vi "Main.vi"(11 "Module Admin":refnum<class "Delacor_lib_QMH_Module Admin.lvclass">) -> ()   [LabVIEW 2020, in "Cycling by Event module.lvlib"]
doc: "This template is based off of the Queued Message Handler design pattern and the Queued Message Handler project template that ships with LabVIEW.\n\nThe main difference is that the queue is private to this module and communication between modules is performed via Broadcast and Request events.\n\nRequest events are wrapped in public API methods and are handled in the Event Handling Loop (EHL) of this VI. Any module can register for Broadcast events sent by this module. The EHL generates messages based on user interface actions.\n\nThe Message Handling Loop (MHL) processes messages generated by the EHL, or by other messages. The messages are string values, so new messages can be added easily to the Message Cases case structure in the MHL. Each message cluster can also provide an optional value for Message Data, which is a variant that can be converted to whatever message-specific data is required.\n_____\nBased on DQMH Project Template 7.0.1.1316."
uses:
  Cycling by Event module.lvlib
  <vilib>/Delacor/Delacor QMH/Libraries/Module Admin_class/Delacor_lib_QMH_Module Admin.lvclass
  Module Data--cluster.ctl
  RPM updated HL Data--cluster.ctl
  Cycling by State module/Cycling state.ctl
  <vilib>/Delacor/Delacor QMH/Libraries/Message Queue_class/Delacor_lib_QMH_Message Queue.lvclass/Delacor_lib_QMH_Message Queue.ctl
  Stop Argument--cluster.ctl
  <vilib>/Delacor/Delacor QMH/Libraries/Module Admin_class/Delacor_lib_QMH_Module Admin.lvclass/Delacor_lib_QMH_Module Admin.ctl
  Start cycling Argument--cluster.ctl
  Detecting 110rpm Argument--cluster.ctl
  Detecting 100rpm Argument--cluster.ctl
  Detecting 0rpm Argument--cluster.ctl
  Stop cycling Argument--cluster.ctl
  <vilib>/Utility/miscctls.llb/LVPointTypeDef.ctl
  <vilib>/Delacor/Delacor QMH/Libraries/Message Queue_class/Delacor_lib_QMH_Enqueue Message (Single).vi
  <vilib>/Delacor/Delacor QMH/Libraries/Module Admin_class/Delacor_lib_QMH_Get External Launch.vi
  <vilib>/Delacor/Delacor QMH/Libraries/Message Queue_class/Delacor_lib_QMH_Message Queue.lvclass
  Sensor checking module/Sensor checking module.lvlib
panel:
  out "error out":errorcluster
  out "Status":string
  in  "Simulate MHL Error":bool
  in  "Simulate EHL Error":bool
  # "Other processes communicate with this Module via its Public API (wrappers for its Request Events).\n\nThis Module communicates with other processes via its Broadcast Events.\nAny process that wants to receive these messages can register for this module's Broadcast events."
  # "This template is for the DQMH framework. See the block diagram for more information on how to use this template."
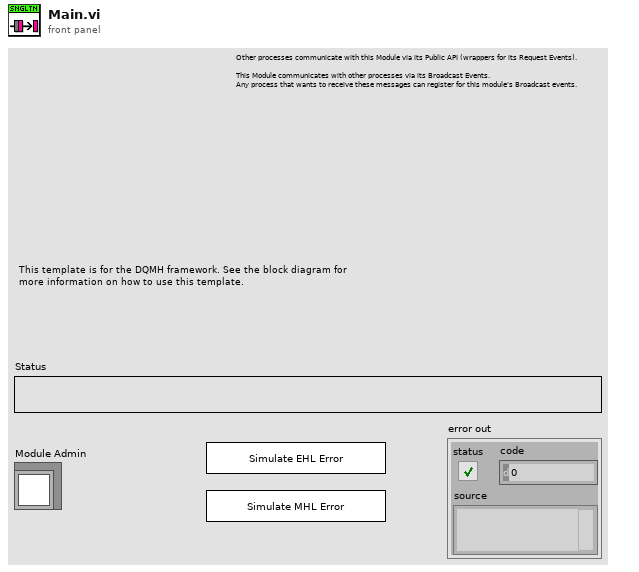
[diagram p1: front panel]
types:
  T1 = typedef "Cycling by Event module.lvlib/Request Events--cluster.ctl" = cluster{"Stop Module":refnum<user-event>, "Show Panel":refnum<user-event>, "Hide Panel":refnum<user-event>, "Get Module Execution Status":refnum<user-event>, "Show Diagram":refnum<user-event>, "Start cycling":refnum<user-event>, "Detecting 110rpm":refnum<user-event>, "Change state to HL":refnum<user-event>, "Detecting 100rpm":refnum<user-event>, "Detecting 0rpm":refnum<user-event>, "Stop cycling":refnum<user-event>}
  T2 = typedef "Sensor checking module.lvlib/Broadcast Events--cluster.ctl" = cluster{"Module Did Init":refnum<user-event>, "Status Updated":refnum<user-event>, "Error Reported":refnum<user-event>, "Module Did Stop":refnum<user-event>, "Update Module Execution Status":refnum<user-event>, "Triggered Broadcast":refnum<user-event>}
  T3 = typedef "Cycling by Event module.lvlib/RPM updated HL Data--cluster.ctl" = cluster{"Enum":T4}
  T4 = typedef "Cycling state.ctl" = enum16{"Accelerating to 110rpm", "Detecting 100rpm", "Pressing until 0rpm"}
  T5 = typedef "Cycling by Event module.lvlib/Module Data--cluster.ctl" = cluster{"Status":string, "Triggered interval":dbl}
  T6 = enum32{"invalid lock state", "Not Locked", "Locked (No Password)", "Password-protected"}
  T7 = typedef "Cycling by Event module.lvlib/Stop Argument--cluster.ctl" = cluster{"Origin":string, "Exit via Stop Module Req?":bool, "Wait for Module to stop?":bool}
  T8 = typedef "Cycling by Event module.lvlib/Start cycling Argument--cluster.ctl" = cluster{"Triggered interval":dbl}
  T9 = typedef "Cycling by Event module.lvlib/Detecting 110rpm Argument--cluster.ctl" = cluster{"RPM":dbl}
  T10 = typedef "Cycling by Event module.lvlib/Detecting 100rpm Argument--cluster.ctl" = cluster{"RPM":dbl}
  T11 = typedef "Cycling by Event module.lvlib/Detecting 0rpm Argument--cluster.ctl" = cluster{"RPM":dbl}
  T12 = typedef "Cycling by Event module.lvlib/Stop cycling Argument--cluster.ctl" = cluster{"Boolean":bool}
  T13 = typedef "LVPointTypeDef.ctl" = cluster{"Horizontal":i16, "Vertical":i16}
  T14 = enum32{"Invalid", "Standard", "Closed", "Hidden", "Minimized", "Maximized"}
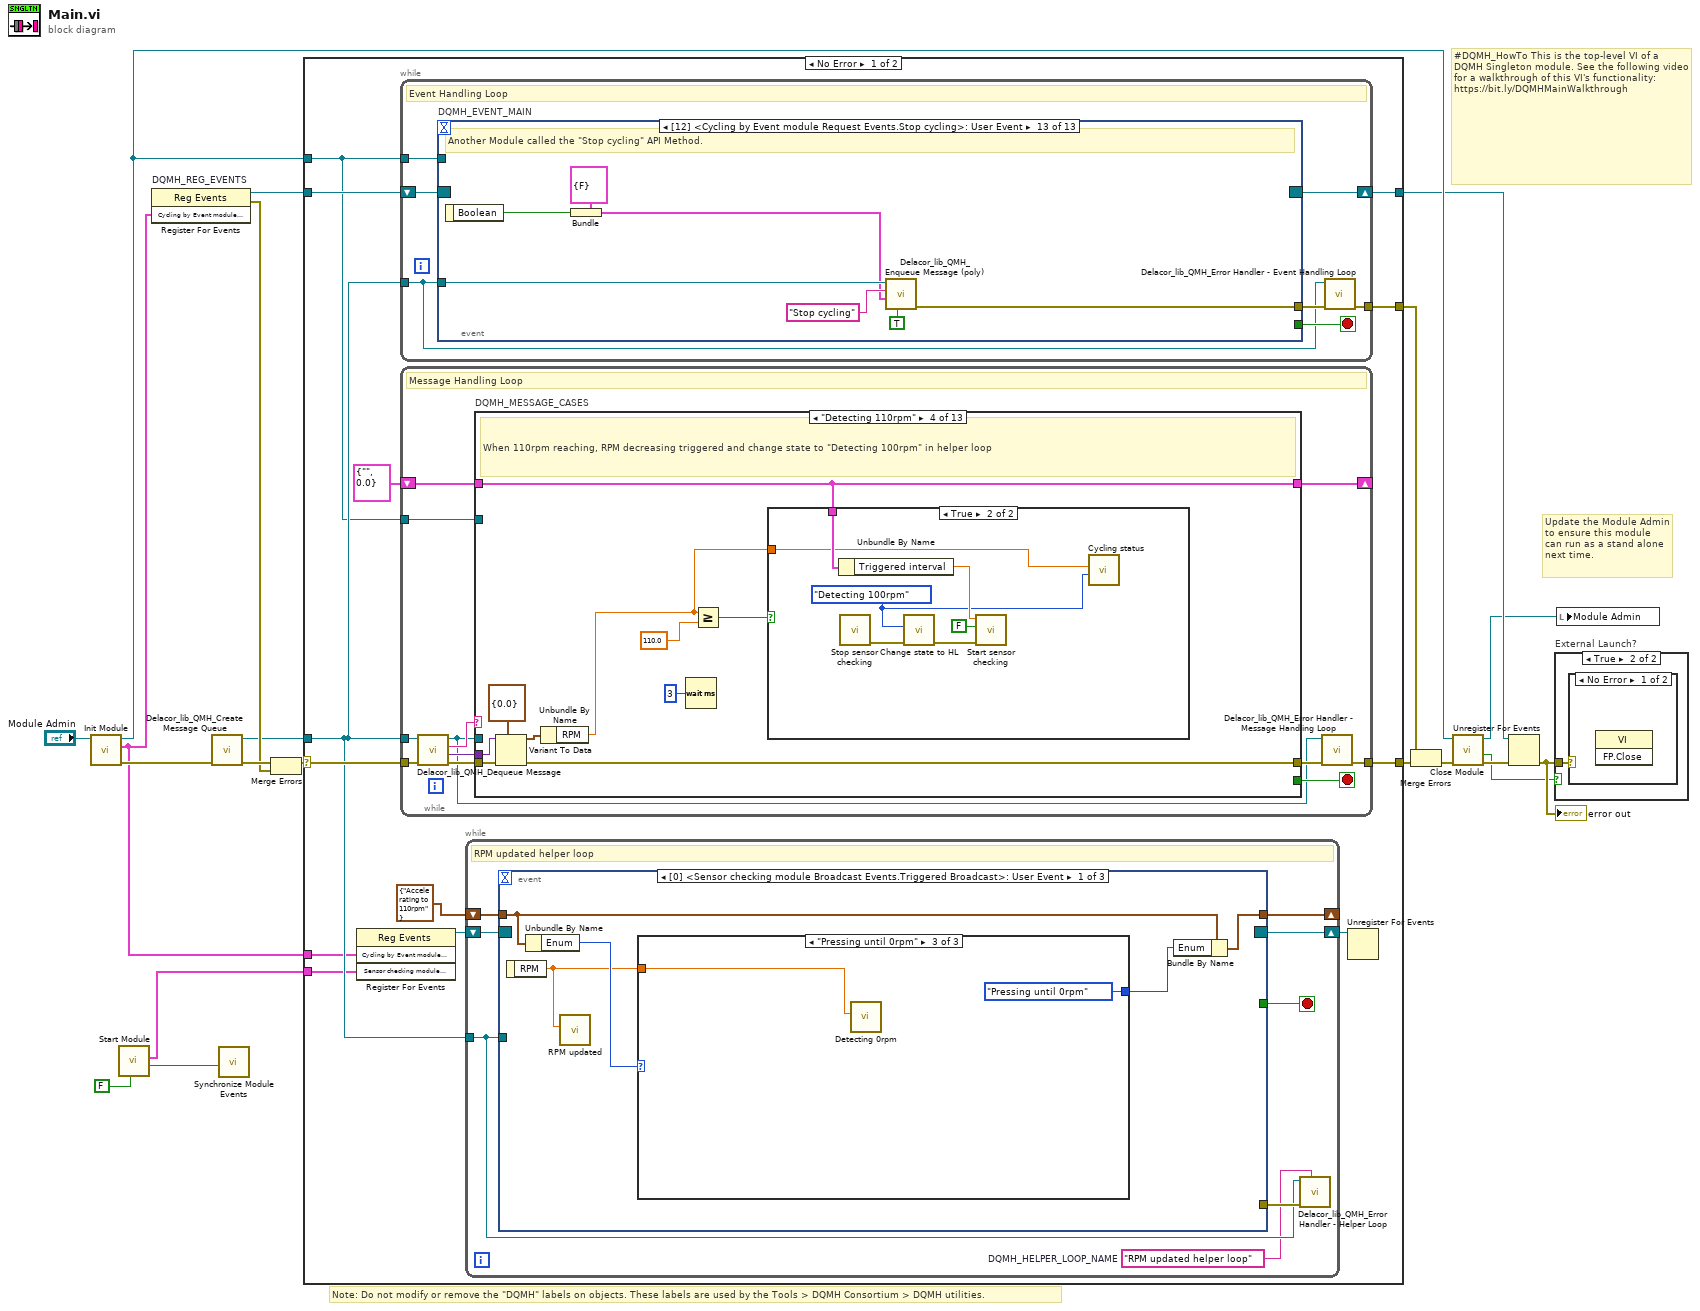
[diagram p0: block diagram]
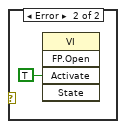
[diagram p3: hidden frame]
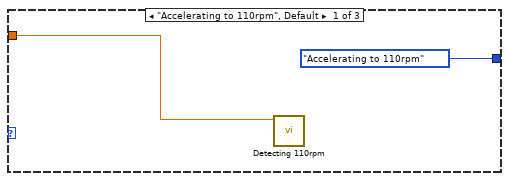
[diagram p4: hidden frame]
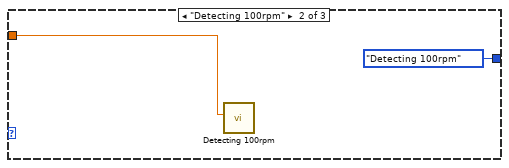
[diagram p5: hidden frame]
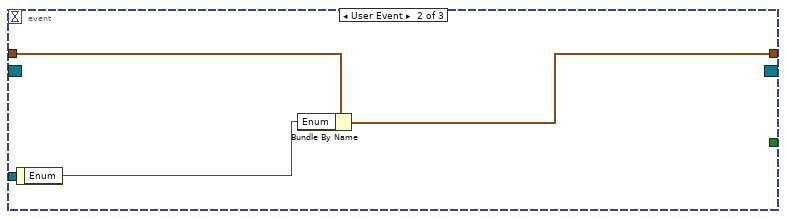
[diagram p6: hidden frame]
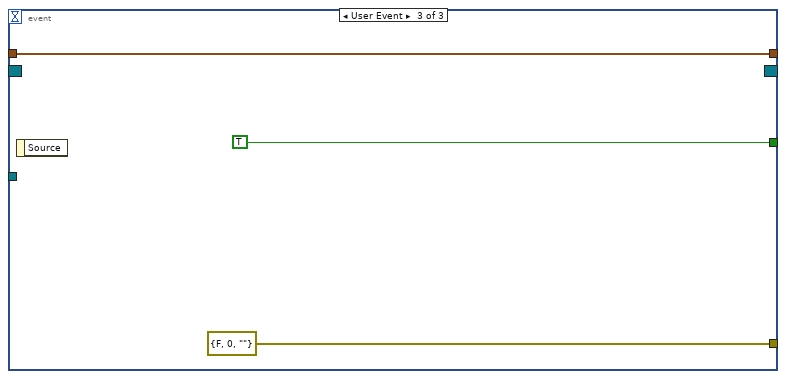
[diagram p7: hidden frame]
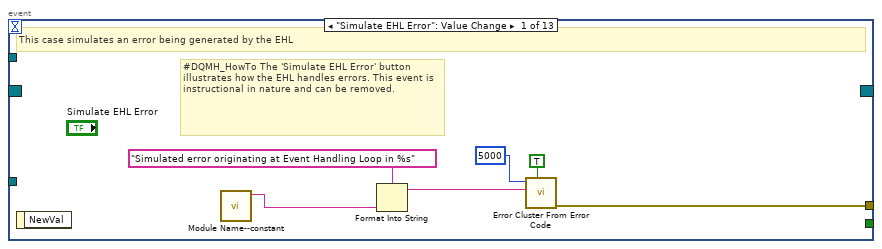
[diagram p8: hidden frame]
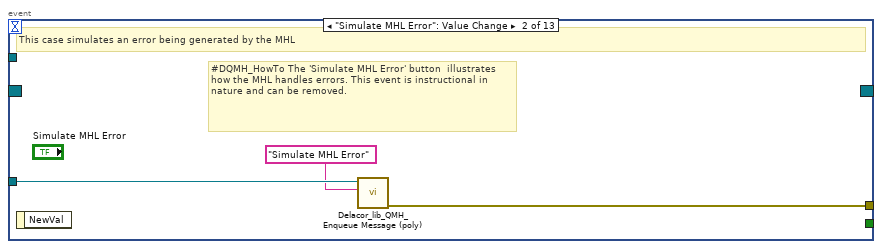
[diagram p9: hidden frame]
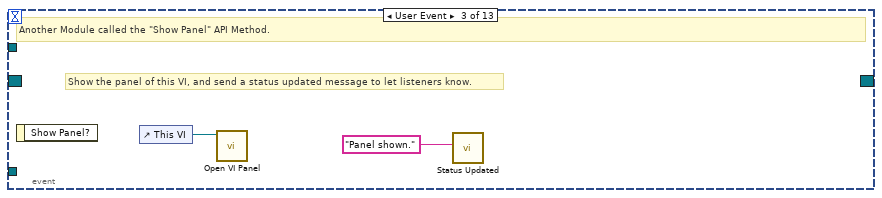
[diagram p10: hidden frame]
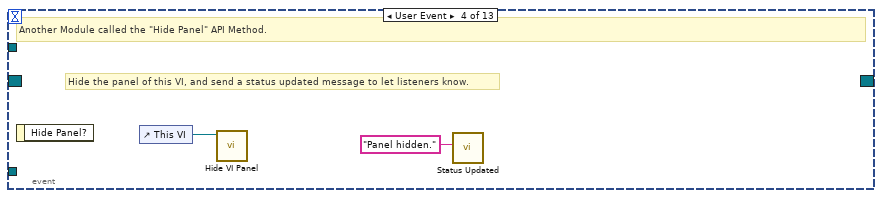
[diagram p11: hidden frame]
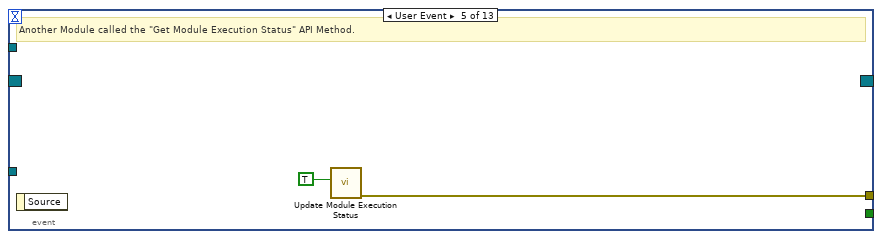
[diagram p12: hidden frame]
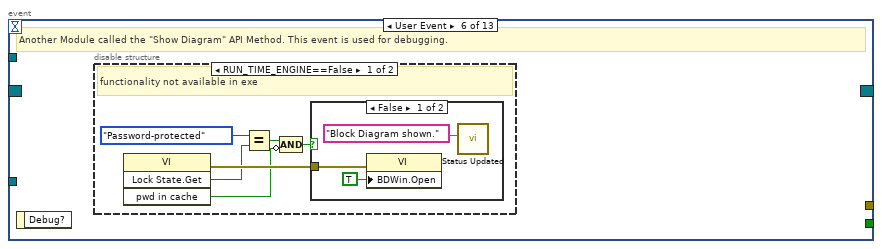
[diagram p13: hidden frame]
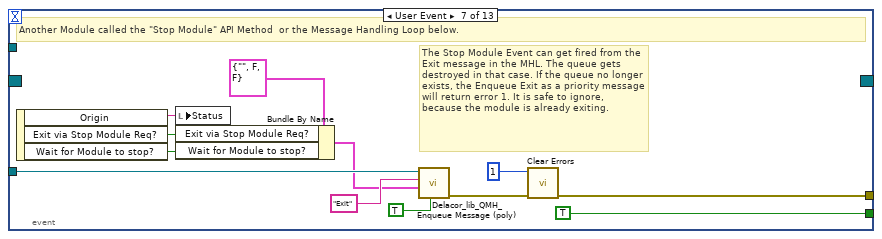
[diagram p16: hidden frame]
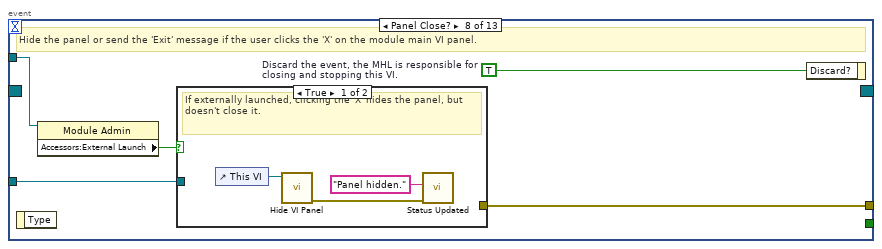
[diagram p17: hidden frame]
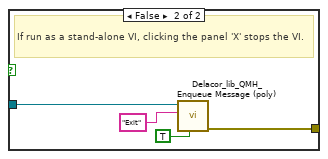
[diagram p18: hidden frame]
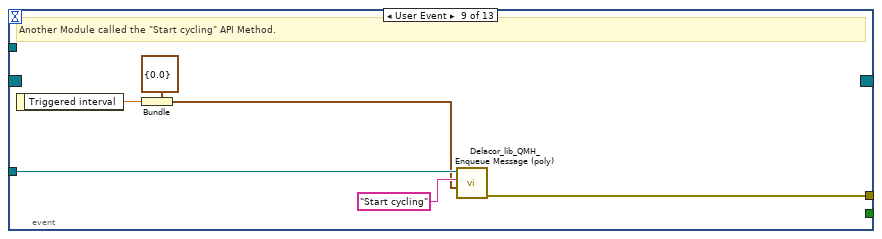
[diagram p19: hidden frame]
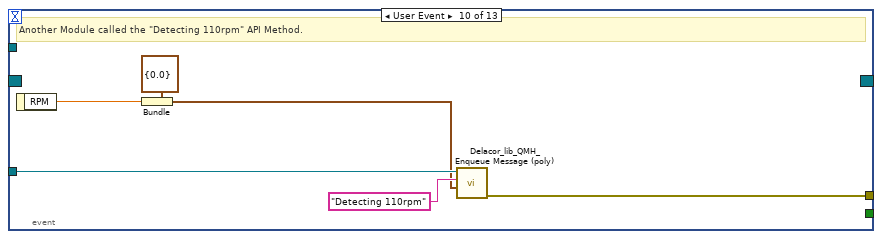
[diagram p20: hidden frame]
diagram:
  # "#DQMH_HowTo This is the top-level VI of a DQMH Singleton module. See the following video for a walkthrough of this VI's functionality: https://bit.ly/DQMHMainWalkthrough"
  # "Note: Do not modify or remove the \"DQMH\" labels on objects. These labels are used by the Tools > DQMH Consortium > DQMH utilities."
  # "Update the Module Admin to ensure this module can run as a stand alone next time."
  n1 = call "Init Module.vi"("Singleton Module Admin in"="Module Admin") -> ("error out"=w19:errorcluster, "Cycling by Event module Request Events"=w4:T1, "Singleton Module Admin out"=w11:refnum<class "Delacor_lib_QMH_Module Admin.lvclass">)  [unwired: 8 in]
  n2 = call "Start Module.vi"("Show Main VI Diagram on Init (F)"=FALSE) -> ("Wait for Event Sync?"=w3:bool, "Sensor checking module Broadcast Events"=w1:T2)  [unwired: 7 in, 2 out]
  n3 = register-events "DQMH_REG_EVENTS"(w4) -> (reference out=w9:refnum<event-registration>, error out=w12:errorcluster)  [unwired: 2 in]
  n4 = call <vilib>:"Delacor_lib_QMH_Create Message Queue.vi"("error in"=w19) -> ("error out"=w14:errorcluster, "Message Queue"=w8:refnum<class "Delacor_lib_QMH_Message Queue.lvclass">)  [unwired: 9 in]
  n5 = call "Synchronize Module Events.vi"("Wait for Event Sync?"=w3) -> ()  [unwired: 10 in, 1 out]
  n6 = Merge Errors(w14, w12) -> (w13:errorcluster)
  n7 = case shown="No Error" w13 {
    selector: w13 -> [w31 w303]
    tunnel: [w33 w302] -> w20
    tunnel: [w30 w301] -> w10
    tunnel: w9 -> [w28 w301]
    tunnel: w8 -> [w27 w296]
    tunnel: [w32 _] -> w17
    tunnel: w11 -> [w26 w297]
    tunnel: w4 -> [w25 _]
    tunnel: w1 -> [w22 _]
    frame No Error {
      n8 = register-events ("DQMH_HELPER_REGFOREVENTS")(w25, w22) -> (reference out=w23:refnum<event-registration>)  [unwired: 2 in, 1 out]
      n9 = while {
        tunnel: w27 -> [w59]
        shift-right: [w62] -> w30
        shift-left: w28 -> [w63]
        tunnel: [w64] -> w32
        tunnel: w26 -> [w60]
        stop <- w61 stop-if-true
        # "Event Handling Loop"
        n10 = event "DQMH_EVENT_MAIN" shown="[12] <Cycling by Event module Request Events.Stop cycling>: User Event" {
          selector: w63 -> [_ _ _ _ _ _ _ _ _ _ _ _ _]
          dyn-events: [_ _ _ _ _ _ _ _ _ _ _ _ _] -> w62
          timeout: _ -> [_ _ _ _ _ _ _ _ _ _ _ _ _]
          tunnel: [_ _ _ _ _ _ TRUE ("Discard?") _ _ _ _ _ _] -> w61
          tunnel: w59 -> [_ w73 _ _ _ _ w97 w104 w119 w125 w131 w137 w144]
          tunnel: [w71 w74 _ _ w80 _ w100 w106 w114 w120 w126 w132 w139] -> w65
          tunnel: w60 -> [_ _ _ _ _ _ _ w103 _ _ _ _ _]
          event "Simulate EHL Error": Value Change {
            # "#DQMH_HowTo The 'Simulate EHL Error' button  illustrates how the EHL handles errors. This event is instructional in nature and can be removed."
            # "This case simulates an error being generated by the EHL"
            n11 = event-data() -> ()  [unwired: 1 in, 1 out]
            n12 = call "Module Name--constant.vi"() -> ("Module Name"=w68:string)  [unwired: 11 in]
            n13 = Format Into String(format string="Simulated error originating at Event Handling Loop in %s", w68) -> (resulting string=w69:string)  [unwired: 2 in, 1 out]
            n14 = call <vilib>:"Error Cluster From Error Code.vi"("show call chain? (False)"=TRUE, "error message (\"\")"=w69, "error code (0)"=5000) -> ("error out"=w71:errorcluster)  [unwired: 6 in]
          }
          event "Simulate MHL Error": Value Change {
            # "#DQMH_HowTo The 'Simulate MHL Error' button  illustrates how the MHL handles errors. This event is instructional in nature and can be removed."
            # "This case simulates an error being generated by the MHL"
            n15 = event-data() -> ()  [unwired: 1 in, 1 out]
            n16 = call-poly <vilib>:"Delacor_lib_QMH_Enqueue Message (poly).vi"("Message"="Simulate MHL Error", "Message Queue in"=w73) -> ("error out"=w74:errorcluster)  [unwired: 8 in, 1 out]
          }
          event User Event {
            # "Show the panel of this VI, and send a status updated message to let listeners know."
            # "Another Module called the \"Show Panel\" API Method."
            n17 = event-data() -> ()  [unwired: 1 in, 1 out]
            n18 = control-ref of="This VI"() -> (w76:refnum<vi>)
            n19 = call "Open VI Panel.vi"("VI"=w76) -> ()  [unwired: 10 in, 1 out]
            n20 = call "Status Updated.vi"("Status"="Panel shown." ("format string")) -> ()  [unwired: 10 in, 1 out]
          }
          event User Event {
            # "Hide the panel of this VI, and send a status updated message to let listeners know."
            # "Another Module called the \"Hide Panel\" API Method."
            n21 = event-data() -> ()  [unwired: 1 in, 1 out]
            n22 = control-ref of="This VI"() -> (w78:refnum<vi>)
            n23 = call "Hide VI Panel.vi"("VI"=w78) -> ()  [unwired: 10 in, 1 out]
            n24 = call "Status Updated.vi"("Status"="Panel hidden." ("format string")) -> ()  [unwired: 10 in, 1 out]
          }
          event User Event {
            # "Another Module called the \"Get Module Execution Status\" API Method."
            n25 = event-data() -> ()  [unwired: 1 in, 1 out]
            n26 = call "Update Module Execution Status.vi"("Running?"=TRUE) -> ("error out"=w80:errorcluster)  [unwired: 10 in]
          }
          event User Event {
            # "Another Module called the \"Show Diagram\" API Method. This event is used for debugging."
            n27 = event-data() -> ()  [unwired: 1 in, 1 out]
            n28 = disable-structure shown="RUN_TIME_ENGINE==False" {
              frame condition #0 (active) {
                # "functionality not available in exe"
                n29 = invoke on="Invoke Node" class="VI" method="Lock State.Get"() -> (error out=w86:errorcluster, "Get Lock State"=w85:T6, "pwd in cache"=w82:bool)  [unwired: 4 in, 1 out]
                n30 = Equal?(x=T6."Password-protected", y=w85) -> (x = y?=w83:bool)
                n31 = Compound Arithmetic op=AND(w83, invert w82) -> (w81:bool)
                n32 = case shown="False" w81 {
                  tunnel: w86 -> [w89 _]
                  frame False {
                    n33 = property on="Property Node" class="VI"(error in=w89, "BDWin.Open"=TRUE ("Block Diagram Window:Open")) -> ()  [unwired: 1 in, 2 out]
                    n34 = call "Status Updated.vi"("Status"="Block Diagram shown." ("format string")) -> ()  [unwired: 10 in, 1 out]
                  }
                  frame True {
                    # "Password-protected VI, and the password is not in the cache. Do not show the diagram."
                  }
                }
              }
              frame condition #1 {
              }
            }
          }
          event User Event {
            # "The Stop Module Event can get fired from the Exit message in the MHL. The queue gets destroyed in that case. If the queue no longer exists, the Enqueue Exit as a priority message will return error 1. It is safe to ignore, because the module is already exiting."
            # "Another Module called the \"Stop Module\" API Method  or the Message Handling Loop below."
            n35 = event-data() -> ("Origin"=w96:string, "Exit via Stop Module Req?"=w92:bool, "Wait for Module to stop?"=w91:bool)  [unwired: 1 in]
            n36 = local write "Status"(w96) -> ()
            n37 = Bundle By Name(cluster=T7 {"Origin"="", "Exit via Stop Module Req?"=FALSE, "Wait for Module to stop?"=FALSE} ("Stop Argument"), "Exit via Stop Module Req?"=w92, "Wait for Module to stop?"=w91) -> (w90:T7)
            n38 = call-poly <vilib>:"Delacor_lib_QMH_Enqueue Message (poly).vi"("Priority Message? (F)"=TRUE, "Message Data"=w90, "Message"="Exit", "Message Queue in"=w97) -> ("error out"=w101:errorcluster)  [unwired: 6 in, 1 out]
            n39 = call <vilib>:"Clear Errors.vi"("error in (no error)"=w101, "specific error code to clear (0: all)"=1) -> ("error out"=w100:errorcluster)  [unwired: 4 in, 1 out]
          }
          event Panel Close? {
            w105 = TRUE  # Discard the event, the MHL is responsible for closing and stopping this VI.
            # "Hide the panel or send the 'Exit' message if the user clicks the 'X' on the module main VI panel."
            n40 = event-data() -> ()  [unwired: 1 in, 1 out]
            n41 = property on="Property Node" class="Module Admin"(reference=w103) -> ("Accessors:External Launch"=w102:bool)  [unwired: 1 in, 2 out]
            n42 = case shown="True" w102 {
              tunnel: w104 -> [_ w112]
              tunnel: [_ w113] -> w106
              frame True {
                # "If externally launched, clicking the 'X' hides the panel, but doesn't close it."
                n43 = control-ref of="This VI"() -> (w109:refnum<vi>)
                n44 = call "Hide VI Panel.vi"("VI"=w109) -> ("error out"=w107:errorcluster)  [unwired: 10 in]
                n45 = call "Status Updated.vi"("error in"=w107, "Status"="Panel hidden." ("format string")) -> ()  [unwired: 9 in, 1 out]
              }
              frame False {
                # "If run as a stand-alone VI, clicking the panel 'X' stops the VI."
                n46 = call-poly <vilib>:"Delacor_lib_QMH_Enqueue Message (poly).vi"("Priority Message? (F)"=TRUE, "Message"="Exit", "Message Queue in"=w112) -> ("error out"=w113:errorcluster)  [unwired: 7 in, 1 out]
              }
            }
            n47 = event-data ("Event Filter Node")("Discard?"=w105) -> ()  [unwired: 1 in, 1 out]
          }
          event User Event {
            # "Another Module called the \"Start cycling\" API Method."
            n48 = event-data() -> ("Triggered interval"=w115:dbl)  [unwired: 1 in]
            n49 = Bundle(cluster=T8 {"Triggered interval"=0.0} ("Start cycling Argument"), "Triggered interval"=w115) -> (w116:T8)
            n50 = call-poly <vilib>:"Delacor_lib_QMH_Enqueue Message (poly).vi"("Message Data"=w116, "Message"="Start cycling", "Message Queue in"=w119) -> ("error out"=w114:errorcluster)  [unwired: 7 in, 1 out]
          }
          event User Event {
            # "Another Module called the \"Detecting 110rpm\" API Method."
            n51 = event-data() -> ("RPM"=w121:dbl)  [unwired: 1 in]
            n52 = Bundle(cluster=T9 {"RPM"=0.0} ("Detecting 110rpm Argument"), "RPM"=w121) -> (w122:T9)
            n53 = call-poly <vilib>:"Delacor_lib_QMH_Enqueue Message (poly).vi"("Message Data"=w122, "Message"="Detecting 110rpm", "Message Queue in"=w125) -> ("error out"=w120:errorcluster)  [unwired: 7 in, 1 out]
          }
          event User Event {
            # "Another Module called the \"Detecting 100rpm\" API Method."
            n54 = event-data() -> ("RPM"=w127:dbl)  [unwired: 1 in]
            n55 = Bundle(cluster=T10 {"RPM"=0.0} ("Detecting 100rpm Argument"), "RPM"=w127) -> (w128:T10)
            n56 = call-poly <vilib>:"Delacor_lib_QMH_Enqueue Message (poly).vi"("Message Data"=w128, "Message"="Detecting 100rpm", "Message Queue in"=w131) -> ("error out"=w126:errorcluster)  [unwired: 7 in, 1 out]
          }
          event User Event {
            # "Another Module called the \"Detecting 0rpm\" API Method."
            n57 = event-data() -> ("RPM"=w133:dbl)  [unwired: 1 in]
            n58 = Bundle(cluster=T11 {"RPM"=0.0} ("Detecting 0rpm Argument"), "RPM"=w133) -> (w134:T11)
            n59 = call-poly <vilib>:"Delacor_lib_QMH_Enqueue Message (poly).vi"("Message Data"=w134, "Message"="Detecting 0rpm", "Message Queue in"=w137) -> ("error out"=w132:errorcluster)  [unwired: 7 in, 1 out]
          }
          event User Event {
            # "Another Module called the \"Stop cycling\" API Method."
            n60 = event-data() -> ("Boolean"=w140:bool)  [unwired: 1 in]
            n61 = Bundle(cluster=T12 {"Boolean"=FALSE} ("Stop cycling Argument"), "Boolean"=w140) -> (w141:T12)
            n62 = call-poly <vilib>:"Delacor_lib_QMH_Enqueue Message (poly).vi"("Priority Message? (F)"=TRUE, "Message Data"=w141, "Message"="Stop cycling", "Message Queue in"=w144) -> ("error out"=w139:errorcluster)  [unwired: 6 in, 1 out]
          }
        }
        n63 = call-dynamic "Delacor_lib_QMH_Error Handler - Event Handling Loop.vi"("error in"=w65, "Message Queue in"=w59) -> ("dup error in"=w64:errorcluster)  [unwired: 8 in, 1 out]
      }
      n64 = while {
        tunnel: w27 -> [w145]
        shift-right: [w153] -> _
        shift-left: T5 {"Status"="", "Triggered interval"=0.0} ("Data Cluster") -> [w154]
        tunnel: w31 -> [w156]
        tunnel: [w148] -> w33
        tunnel: w26 -> [w149]
        stop <- w152 stop-if-true
        # "Message Handling Loop"
        n65 = call-dynamic "Delacor_lib_QMH_Dequeue Message.vi"("error in"=w156, "Message Queue in"=w145) -> ("error out"=w155:errorcluster, "Message Data"=w150:variant, "Message"=w151:string, "Message Queue out"=w146:refnum<class "Delacor_lib_QMH_Message Queue.lvclass">)  [unwired: 6 in]
        n66 = case "DQMH_MESSAGE_CASES" shown="\"Detecting 110rpm\"" w151 {
          selector: w151 -> [_ _ _ _ _ _ _ _ _ _ _ _ w291]
          tunnel: w146 -> [_ _ _ _ _ _ _ _ _ _ w257 w279 _]
          tunnel: w155 -> [w174 w178 w189 w199 w215 w226 w239 w242 w244 w253 w264 w285 w294]
          tunnel: [w172 w178 w188 w198 w214 w225 w237 w241 w244 w252 w260 w280 w295] -> w147
          tunnel: w154 -> [w163 w177 w181 w192 w208 w219 w238 w240 w243 w250 w259 w278 w292]
          tunnel: [w162 w177 w180 w192 w208 w219 w238 w240 w243 w250 w259 w278 w292] -> w153
          tunnel: [_ _ _ _ _ _ _ _ _ _ _ w277 _] -> w152
          tunnel: w150 -> [_ _ w187 w197 w213 w224 w236 _ _ _ w258 w276 _]
          tunnel: w149 -> [w164 _ _ _ _ _ _ _ _ _ w256 w271 _]
          frame "Initialize" {
            w158 = "Initial Message" ("Initial Message")
            # "#CodeNeeded - Initialize the appearance of the front panel."
            # "#CodeNeeded - Initialize your state data here."
            # "Initialize - Any operation that needs to be done before the module can receive messages. Synchronize Caller Events.vi will inform Start Module.vi that the module has launched and is ready to receive messages. Module Did Init.vi will broadcast that the module initialized."
            n67 = call "Synchronize Caller Events.vi"("error in"=w174, "Singleton Module Admin in"=w164) -> ("error out"=w173:errorcluster, "Singleton Module Admin out"=w159:refnum<class "Delacor_lib_QMH_Module Admin.lvclass">)  [unwired: 8 in]
            n68 = property on="Property Node" class="Module Admin"(reference=w159) -> ("Accessors:External Launch"=w168:bool)  [unwired: 1 in, 2 out]
            n69 = Select(t=T14."Hidden" ("State"), s=w168, f=T14."Standard" ("State")) -> (s? t:f=w165:T14)
            n70 = call "Module Name--constant.vi"() -> ("Module Name"=w171:string)  [unwired: 11 in]
            n71 = property on="Property Node" class="VI"("Front Panel.Title"=w171) -> (reference out=w170:refnum<vi>, error out=w176:errorcluster)  [unwired: 2 in]
            n72 = call "Module Name--constant.vi"() -> ("Module Name"=w160:string)  [unwired: 11 in]
            n73 = invoke on="Invoke Node" class="VI" method="FP.Open"(reference=w170, error in=w176, "State"=w165) -> (reference out=w169:refnum<vi>, error out=w175:errorcluster)  [unwired: 2 in, 3 out]
            n74 = Bundle By Name(cluster=w163, "Status"=w158) -> (w162:T5)
            n75 = call "Module Did Init.vi"("error in"=w173, "Initialized?"=TRUE, "Origin"=w160) -> ("error out"=w172:errorcluster)  [unwired: 8 in]
            n76 = invoke on="Invoke Node" class="VI" method="FP.Center"(reference=w169, error in=w175) -> ()  [unwired: 1 in, 3 out]
            n77 = property on="Pane" class="Pane"("Origin"=T13 {"Horizontal"=0, "Vertical"=0}) -> ()  [unwired: 2 in, 2 out]
            "Status" <- w158
          }
          frame "---Module Specific---" {
            # "Separator -- The following cases handle messages specific to this Module."
          }
          frame "Start cycling" {
            # "Start Sensor checking module to revieve RPM broadcast"
            n78 = Variant To Data(error in=w189, type=T8 {"Triggered interval"=0.0} ("Start cycling Argument"), Variant=w187) -> (data=w185:T8, error out=w188:errorcluster)
            n79 = Unbundle By Name(w185) -> ("Triggered interval"=w179:dbl)
            n80 = Bundle By Name(cluster=w181, "Triggered interval"=w179) -> (w180:T5)
            n81 = call "Change state to HL.vi"("Enum"=Cycling_state."Accelerating to 110rpm") -> ("error out"=w183:errorcluster)  [unwired: 10 in]
            n82 = call "Start sensor checking.vi"("Triggered interval"=w179, "RPM increasing?"=TRUE, "error in"=w183) -> ()  [unwired: 7 in, 1 out]
          }
          frame "Detecting 110rpm" {
            # "When 110rpm reaching, RPM decreasing triggered and change state to \"Detecting 100rpm\" in helper loop"
            n83 = Variant To Data(error in=w199, type=T9 {"RPM"=0.0} ("Detecting 110rpm Argument"), Variant=w197) -> (data=w195:T9, error out=w198:errorcluster)
            n84 = Unbundle By Name(w195) -> ("RPM"=w191:dbl)
            n85 = Wait (ms)(milliseconds to wait=u32 3) -> ()  [unwired: 1 out]
            n86 = Greater Or Equal?(x=w191, y=110.0) -> (x >= y?=w194:bool)
            n87 = case shown="True" w194 {
              tunnel: w192 -> [_ w205]
              tunnel: w191 -> [_ w201]
              frame False {
              }
              frame True {
                w200 = Cycling_state."Detecting 100rpm" ("Enum")
                n88 = Unbundle By Name(w205) -> ("Triggered interval"=w204:dbl)
                n89 = call "Stop sensor checking.vi"() -> ("error out"=w203:errorcluster)  [unwired: 11 in]
                n90 = call "Change state to HL.vi"("error in"=w203, "Enum"=w200) -> ("error out"=w202:errorcluster)  [unwired: 9 in]
                n91 = call "Start sensor checking.vi"("Triggered interval"=w204, "RPM increasing?"=FALSE, "error in"=w202) -> ()  [unwired: 7 in, 1 out]
                n92 = call "Cycling status.vi"("Enum"=w200, "RPM"=w201) -> ()  [unwired: 9 in, 1 out]
              }
            }
          }
          frame "Detecting 100rpm" {
            # "When 100rpm reaching, change state to \"Pressing until 0rpm\" in helper loop"
            n93 = Variant To Data(error in=w215, type=T10 {"RPM"=0.0} ("Detecting 100rpm Argument"), Variant=w213) -> (data=w211:T10, error out=w214:errorcluster)
            n94 = Unbundle By Name(w211) -> ("RPM"=w207:dbl)
            n95 = Less Or Equal?(x=w207, y=100.0) -> (x <= y?=w210:bool)
            n96 = case shown="True" w210 {
              tunnel: w207 -> [_ w217]
              frame False {
              }
              frame True {
                w216 = Cycling_state."Pressing until 0rpm" ("Enum")
                n97 = call "Change state to HL.vi"("Enum"=w216) -> ()  [unwired: 10 in, 1 out]
                n98 = call "Cycling status.vi"("Enum"=w216, "RPM"=w217) -> ()  [unwired: 9 in, 1 out]
              }
            }
          }
          frame "Detecting 0rpm" {
            # "When 0rpm reaching, change state to \"Accelerating to 110rpm\" in helper loop for next cycle"
            n99 = Variant To Data(error in=w226, type=T11 {"RPM"=0.0} ("Detecting 0rpm Argument"), Variant=w224) -> (data=w222:T11, error out=w225:errorcluster)
            n100 = Unbundle By Name(w222) -> ("RPM"=w218:dbl)
            n101 = Less Or Equal?(x=w218, y=0.0) -> (x <= y?=w221:bool)
            n102 = case shown="True" w221 {
              tunnel: w219 -> [_ w232]
              tunnel: w218 -> [_ w228]
              frame False {
              }
              frame True {
                w227 = Cycling_state."Accelerating to 110rpm" ("Enum")
                n103 = Unbundle By Name(w232) -> ("Triggered interval"=w231:dbl)
                n104 = call "Stop sensor checking.vi"() -> ("error out"=w230:errorcluster)  [unwired: 11 in]
                n105 = call "Change state to HL.vi"("error in"=w230, "Enum"=w227) -> ("error out"=w229:errorcluster)  [unwired: 9 in]
                n106 = call "Start sensor checking.vi"("Triggered interval"=w231, "RPM increasing?"=TRUE, "error in"=w229) -> ()  [unwired: 7 in, 1 out]
                n107 = call "Cycling status.vi"("Enum"=w227, "RPM"=w228) -> ()  [unwired: 9 in, 1 out]
              }
            }
          }
          frame "Stop cycling" {
            # "Stop cycling by stopping sensor detecting"
            n108 = Variant To Data(error in=w239, type=T12 {"Boolean"=FALSE} ("Stop cycling Argument"), Variant=w236) -> (data=w234:T12, error out=w237:errorcluster)
            n109 = Unbundle By Name(w234) -> ()  [unwired: 1 out]
            n110 = call "Stop sensor checking.vi"() -> ()  [unwired: 11 in, 1 out]
          }
          frame "---Copy This Frame---" {
            # "Duplicate this frame when creating new messages.  Change this comment in the duplicated frame to describe this message."
            n111 = Merge Errors(w242) -> (w241:errorcluster)
          }
          frame "---Exit and Error Handling---" {
            # "Separator - The following cases handle errors and exit messages."
          }
          frame "Simulate MHL Error" {
            # "#DQMH_HowTo The 'Simulate MHL Error' button  illustrates how the MHL handles errors. This event is instructional in nature and can be removed."
            # "Simulate an error occurring at the MHL"
            n112 = call "Module Name--constant.vi"() -> ("Module Name"=w246:string)  [unwired: 11 in]
            n113 = Format Into String(format string="Simulated error originating at Message Handling Loop in %s", w246) -> (resulting string=w247:string)  [unwired: 2 in, 1 out]
            n114 = call <vilib>:"Error Cluster From Error Code.vi"("show call chain? (False)"=TRUE, "error message (\"\")"=w247, "error code (0)"=5001) -> ("error out"=w251:errorcluster)  [unwired: 6 in]
            n115 = Merge Errors(w253, w251) -> (w252:errorcluster)
          }
          frame "Error" {
            # "#CodeRecommended - If the module is running in standalone mode (External Launch = FALSE), this code will pop up an error dialog and call the 'Exit' message if an error occurs. Add more fine-grained error management here."
            # "Error - Check the error message data and respond accordingly. This message is sent by the \"Error Handler\" VIs at the end of each loop in this application."
            n116 = property on="Property Node" class="Module Admin"(reference=w256) -> ("Accessors:External Launch"=w255:bool)  [unwired: 1 in, 2 out]
            n117 = Variant To Data(error in=w264, type=errorcluster {"status"=FALSE, "code"=0, "source"=""} ("error constant"), Variant=w258) -> (data=w254:errorcluster, error out=w262:errorcluster)
            n118 = local write "error out"(w254) -> ()
            n119 = call "Error Reported.vi"("Error"=w254) -> ()  [unwired: 10 in, 1 out]
            n120 = case shown="False" w255 {
              tunnel: [w269 _] -> w261
              tunnel: w257 -> [w267 _]
              tunnel: w254 -> [w268 _]
              frame False {
                n121 = disable-structure shown="Default" {
                  disable-tunnel: w268 -> [w270 _]
                  frame condition #0 (active) {
                    # "If the module is running standalone, then pop up an error dialog and call the \"Exit\" message."
                    n122 = call <vilib>:"Simple Error Handler.vi"("error in (no error)"=w270) -> ()  [unwired: 4 in, 5 out]
                  }
                  frame condition #1 {
                    # "To prevent the Simple Error Handler VI from being loaded (e.g. when deploying to a Real-Time target), add the Conditional Disable Symbol \"DQMH_Disable_SEH\" to your project and set it to TRUE."
                  }
                }
                n123 = call-poly <vilib>:"Delacor_lib_QMH_Enqueue Message (poly).vi"("Priority Message? (F)"=TRUE, "Message"="Exit", "Message Queue in"=w267) -> ("error out"=w269:errorcluster)  [unwired: 7 in, 1 out]
              }
              frame True {
                # "If the module was launched externally, calling the Error Reported broadcast VI is the only action performed by the \"Error\" message. The module's caller can then process the error appropriately."
              }
            }
            n124 = Merge Errors(w262, w261) -> (w260:errorcluster)
          }
          frame "Exit" {
            w275 = 91  # 91: not all Exit messages will have an argument
            w277 = TRUE  # Stop the VI
            # "Release the message queue reference"
            # "#CodeNeeded - Add any required cleanup code here."
            # "Exit - Exit the application."
            n125 = Variant To Data(error in=w285, type=T7 {"Origin"="", "Exit via Stop Module Req?"=FALSE, "Wait for Module to stop?"=FALSE} ("Stop Argument"), Variant=w276) -> (data=w273:T7, error out=w282:errorcluster)
            n126 = call <vilib>:"Clear Errors.vi"("error in (no error)"=w282, "specific error code to clear (0: all)"=w275) -> ("error out"=w284:errorcluster)  [unwired: 4 in, 1 out]
            n127 = control-ref of="This VI"() -> (w272:refnum<vi>)
            n128 = call-dynamic "Delacor_lib_QMH_Release Message Queue.vi"("error in"=w284, "Message Queue"=w279) -> ("error out"=w283:errorcluster)  [unwired: 9 in]
            n129 = call "Handle Exit.vi"("Stop Argument"=w273, "Admin in"=w271, "VI reference"=w272) -> ("error out"=w281:errorcluster)  [unwired: 7 in, 1 out]
            n130 = Merge Errors(w283, w281) -> (w280:errorcluster)
            n131 = call "Error Reported.vi"("Error"=w280) -> ()  [unwired: 10 in, 1 out]
            n132 = call "Stop Module.vi"() -> ()  [unwired: 11 in, 1 out]
          }
          frame Default {
            # "'Default' case only runs if there is a message that isn't defined in any of the other cases.  Output a programming error."
            n133 = call "Module Name--constant.vi"() -> ("Module Name"=w290:string)  [unwired: 11 in]
            n134 = Format Into String(format string="The invalid message string \"%s\" was received in the Message Handling Loop for module \"%s\".", w291, w290) -> (resulting string=w286:string)  [unwired: 2 in, 1 out]
            n135 = call <vilib>:"Error Cluster From Error Code.vi"("show call chain? (False)"=TRUE, "error message (\"\")"=w286, "error code (0)"=1) -> ("error out"=w293:errorcluster)  [unwired: 6 in]
            n136 = Merge Errors(w294, w293) -> (w295:errorcluster)
          }
        }
        n137 = call-dynamic "Delacor_lib_QMH_Error Handler - Message Handling Loop.vi"("error in"=w147, "Message Queue in"=w146) -> ("dup error in"=w148:errorcluster)  [unwired: 8 in, 1 out]
      }
      n138 = while "DQMH_HELPER_LOOP" {
        shift-right: [w40] -> w24
        shift-left: w23 -> [w41]
        tunnel: w27 -> [w37]
        shift-right: [w34] -> _
        shift-left: T3 {"Enum"=enum."Accelerating to 110rpm"} ("RPM updated HL Data") -> [w35]
        stop <- w39 stop-if-true
        w36 = "RPM updated helper loop"  # DQMH_HELPER_LOOP_NAME
        # "RPM updated helper loop"
        n139 = event "DQMH_HELPER_EVENT_STRUCTURE" shown="[0] <Sensor checking module Broadcast Events.Triggered Broadcast>: User Event" {
          selector: w41 -> [_ _ _]
          dyn-events: [_ _ _] -> w40
          timeout: _ -> [_ _ _]
          tunnel: [_ _ TRUE] -> w39
          tunnel: [_ _ errorcluster {"status"=FALSE, "code"=0, "source"=""} ("error constant")] -> w38
          tunnel: w37 -> [_ _ _]
          tunnel: w35 -> [w45 w55 w56]
          tunnel: [w44 w54 w56] -> w34
          event User Event {
            n140 = event-data() -> ("RPM"=w42:dbl)  [unwired: 1 in]
            n141 = Unbundle By Name(w45) -> ("Enum"=w46:T4)
            n142 = call "RPM updated.vi"("RPM"=w42) -> ()  [unwired: 10 in, 1 out]
            n143 = case shown="\"Pressing until 0rpm\"" w46 {
              tunnel: [Cycling_state."Accelerating to 110rpm" ("Enum") Cycling_state."Detecting 100rpm" ("Enum") Cycling_state."Pressing until 0rpm" ("Enum")] -> w43
              tunnel: w42 -> [w47 w49 w52]
              frame "Accelerating to 110rpm", Default {
                n144 = call "Detecting 110rpm.vi"("RPM"=w47) -> ()  [unwired: 10 in, 1 out]
              }
              frame "Detecting 100rpm" {
                n145 = call "Detecting 100rpm.vi"("RPM"=w49) -> ()  [unwired: 10 in, 1 out]
              }
              frame "Pressing until 0rpm" {
                n146 = call "Detecting 0rpm.vi"("RPM"=w52) -> ()  [unwired: 10 in, 1 out]
              }
            }
            n147 = Bundle By Name(cluster=w45, "Enum"=w43) -> (w44:T3)
          }
          event User Event {
            n148 = event-data() -> ("Enum"=w53:T4)  [unwired: 1 in]
            n149 = Bundle By Name(cluster=w55, "Enum"=w53) -> (w54:T3)
          }
          event User Event {
            n150 = event-data() -> ()  [unwired: 1 in, 1 out]
          }
        }
        n151 = call-dynamic "Delacor_lib_QMH_Error Handler - Helper Loop.vi"("Error Debug"=w36, "error in"=w38, "Message Queue in"=w37) -> ()  [unwired: 7 in, 2 out]
      }
      n152 = Unregister For Events(event registration refnum=w24) -> ()  [unwired: 1 in, 1 out]
    }
    frame Error {
      # "Synchronize Caller Events.vi will inform Start Module.vi that the module has launched and will let the code calling Start Module.vi register for broadcasts and would permit the caller receive the broadcast that an error occurred at launch time."
      n153 = call-dynamic "Delacor_lib_QMH_Release Message Queue.vi"("error in"=w303, "Message Queue"=w296) -> ("error out"=w302:errorcluster)  [unwired: 9 in]
      n154 = call "Synchronize Caller Events.vi"("Singleton Module Admin in"=w297) -> ("error out"=w304:errorcluster)  [unwired: 9 in, 1 out]
      n155 = call "Module Name--constant.vi"() -> ("Module Name"=w300:string)  [unwired: 11 in]
      n156 = Format Into String(format string="An error occurred during initialization. %s is no longer running.", w300) -> (resulting string=w298:string)  [unwired: 2 in, 1 out]
      n157 = Merge Errors(w302, w304) -> (w305:errorcluster)
      n158 = call "Error Reported.vi"("Additional Information"=w298, "Error"=w305) -> ()  [unwired: 9 in, 1 out]
    }
  }
  n159 = Merge Errors(w17, w20) -> (w16:errorcluster)
  n160 = call "Close Module.vi"("error in"=w16, "Module Admin in"=w11) -> ("error out"=w18:errorcluster, "External Launch"=w5:bool, "Module Admin out"=w6:refnum<class "Delacor_lib_QMH_Module Admin.lvclass">)  [unwired: 7 in]
  n161 = Unregister For Events(event registration refnum=w10, error in=w18) -> (error out=w15:errorcluster)
  "error out" <- w15
  n162 = case "External Launch?" shown="True" w5 {
    tunnel: w15 -> [_ w306]
    frame False {
    }
    frame True {
      n163 = case shown="No Error" w306 {
        frame No Error {
          n164 = invoke on="Invoke Node" class="VI" method="FP.Close"() -> ()  [unwired: 3 in, 3 out]
        }
        frame Error {
          n165 = invoke on="Invoke Node" class="VI" method="FP.Open"("Activate"=TRUE ("Activate?")) -> ()  [unwired: 4 in, 5 out]
        }
      }
    }
  }
  n166 = local write "Module Admin"(w6) -> ()
